vi "Merc_Connection_Example.vi"(0 "VISA resource name":refnum<visa-resource-name>, 1 "IP Address":string, 5 "Comms Layer":T1, 7 "Serial Configuration":T3={"Baud Rate"=9600, "Parity"=0, "Data Bits"=8, "Stop Bits"=10, "Flow Control"=0} {"Flow Control" items=["None", "XON/XOFF", "RTS/CTS", "XON/XOFF & RTS/CTS", "DTR/DSR", "XON/XOFF & DTR/DSR"]; "Stop Bits" items=["1.0"=10, "2.0"=20]; "Data Bits" items=["7"=7, "8"=8]; "Parity" items=["None", "Odd", "Even"]; "Baud Rate" items=["300"=300, "600"=600, "1200"=1200, "2400"=2400, "4800"=4800, "9600"=9600, "19200"=19200]}, 9 "ID Query (True)":bool, 11 "error in (no error)":errorcluster, 12 "Clear Previous Connections (False)":bool, 13 "ISOBUS address":T2=-1 caption="ISOBUS address (-1)") -> (3 "Devices":string[](array[string]), 4 "Mercury Reference Out":T5, 6 "# of Instruments":i32, 8 "S/W Version(s)":string[](array[string]), 10 "Serial Number(s)":string[](array[string]), 14 "Valid?":T4, 15 "error out":errorcluster)   [LabVIEW 2016, in "Mercury iXX.lvlib"]
uses:
  Mercury iXX.lvlib
  Public/Controls/Comms Transport Layer.ctl
  Public/Controls/Serial Settings.ctl
  Public/Controls/ISOBus Address.ctl
  Public/Controls/Is Valid LED.ctl
  Public/Controls/Mercury Reference.ctl
  Private/Controls/Query Dynamic Reference.ctl
  Public/Libraries/System/Open/Open System.vi
  Public/Libraries/System/Read/Catalogue (Read).vi
  Public/Libraries/System.lvlib
panel:
  in  "Tab Control":enum32{"Connection", "Devices"}(tab)
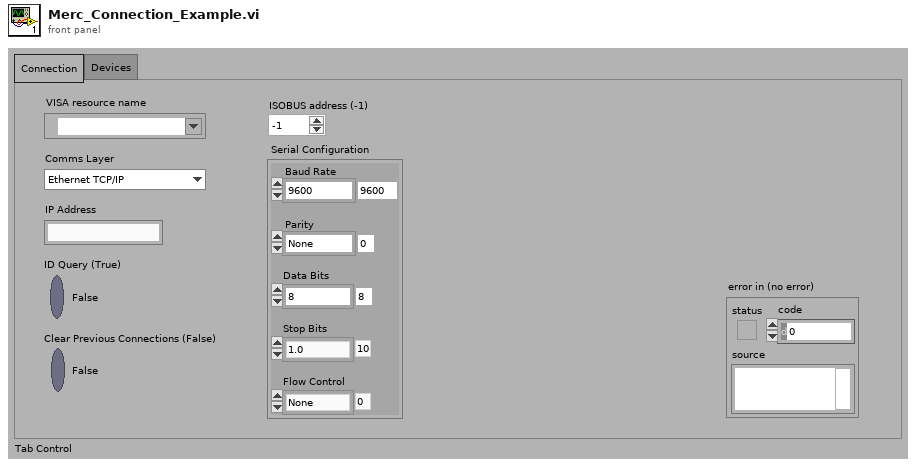
[diagram p1: front panel]
types:
  T1 = typedef "Mercury iXX.lvlib/Comms Transport Layer.ctl" = enum16{"Ethernet TCP/IP", "USB", "ISOBus - RS-232", "GPIB"}
  T2 = typedef "Mercury iXX.lvlib/ISOBus Address.ctl" = i32
  T3 = typedef "Mercury iXX.lvlib/Serial Settings.ctl" = cluster{"Baud Rate":u32, "Parity":u16, "Data Bits":u16, "Stop Bits":u16, "Flow Control":u16}
  T4 = typedef "Mercury iXX.lvlib/Is Valid LED.ctl" = bool
  T5 = typedef "Mercury iXX.lvlib/Mercury Reference.ctl" = cluster{"Comms":refnum<visa-resource-name>, "Device ID":string[], "Comms Layer":T1, "Command":string, "Query reference":T6}
  T6 = typedef "Mercury iXX.lvlib/Query Dynamic Reference.ctl" = refnum<vi>
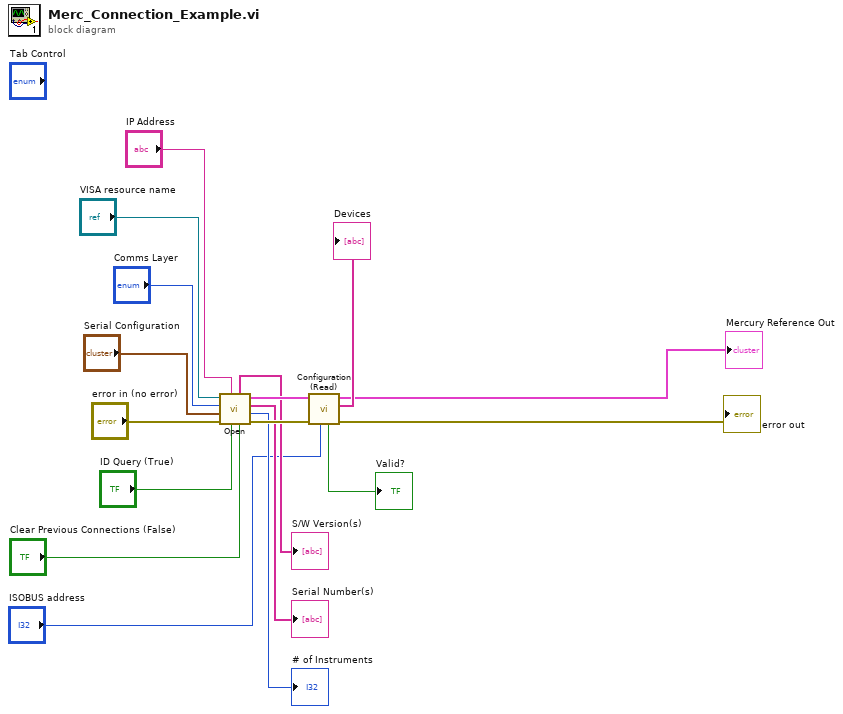
[diagram p0: block diagram]
diagram:
  n1 = call-poly "Open.vi"("Clear Previous Connections (False)"="Clear Previous Connections (False)", "ID Query (True)"="ID Query (True)", "IP Address"="IP Address", "error in (no error)"="error in (no error)", "Serial Configuration"="Serial Configuration", "Comms Layer"="Comms Layer", "VISA resource name"="VISA resource name") -> ("error out"=w16:errorcluster, "# of Instruments"=→"# of Instruments":i32, "Serial Number(s)"=→"Serial Number(s)":string[], "Mercury Reference Out"=w17:T5, "S/W Version(s)"=→"S/W Version(s)":string[])
  n2 = call-poly "Configuration (Read).vi"("ISOBUS address"="ISOBUS address", "error in"=w16, "Mercury Reference In"=w17) -> ("error out"=→"error out":errorcluster, "Devices"=→"Devices":string[], "Mercury Reference Out"=→"Mercury Reference Out":T5, "Valid?"=→"Valid?":T4)  [unwired: 5 out]
